vi "IKGMS.vi"(0 "delimiter (Tab)":string="\t", 1 "transpose? (no:F)":bool, 4 "format (%.3f)":string="%.2f", 5 "append to file? (new file:F)":bool, 6 "1D data":sgl[](array[numeric]) format="%.2f", 7 "2D data":sgl[][](array[numeric]) format="%.2f", 8 "file path (dialog if empty)":path) -> (3 "new file path (Not A Path if cancelled)":path)   [LabVIEW 2016]
doc: "Converts a 2D or 1D array of single-precision numbers to a text string and writes the string to a new byte stream file or appends the string to an existing file. You can optionally transpose the data. This VI opens or creates the file beforehand and closes it afterwards. You can use this VI to create a text file readable by most spreadsheet applications.\n\nfile path is the path name of the file. If file path is empty (default value) or is Not A Path, the VI displays a File dialog box from which you can select a file. Error 43 occurs if the user cancels the dialog. \n\n2D data contains the single-precision numbers the VI writes to the file if 1D data is not wired or is empty.\n\n1D data contains the single-precision numbers the VI writes to the file if this input is not empty. The VI converts the 1D array into a 2D array before transposing it and converting it to a string and writing it to the file. If transpose? is FALSE, each call to this VI creates a new line or row in the file.\n\nappend to file? Set to TRUE if you want to append the data to a existing file; you can also set it TRUE to write to a new file. Set to FALSE (default value) if you want to write the data to a new file or to replace an existing file. \n\ntranspose? Set TRUE to transpose the data before converting it to a string. The default value is FALSE.\n\nformat specifies how to convert the numbers to characters. If the format string is %.3f (default), the VI creates a string long enough to contain the number, with three digits to the right of the decimal point. If the format is %d, the VI converts the data to integer form using as many characters as necessary to contain the entire number. Refer to the discussion of format strings and the Array To Spreadsheet String function in Chapter 6, String Functions, of the LabVIEW Function Reference Manual.\n\nnew file path is the path of the file to which the VI wrote data. You can use this output to determine the path of a file that you open using dialog. new file path returns Not A Path if the user selects Cancel from the dialog box."
uses:
  ad interface/Global_SIM_switch.vi
  utilities/numrowglobal.vi
panel:
  out "NUMROWS Read":dbl format="%.2f"
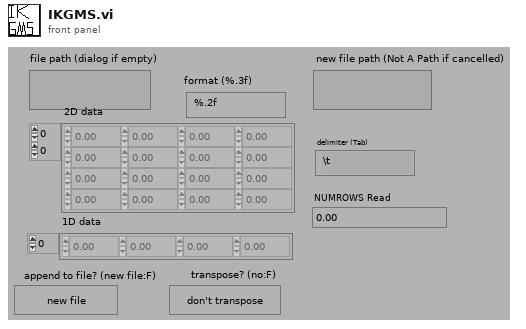
[diagram p1: front panel]
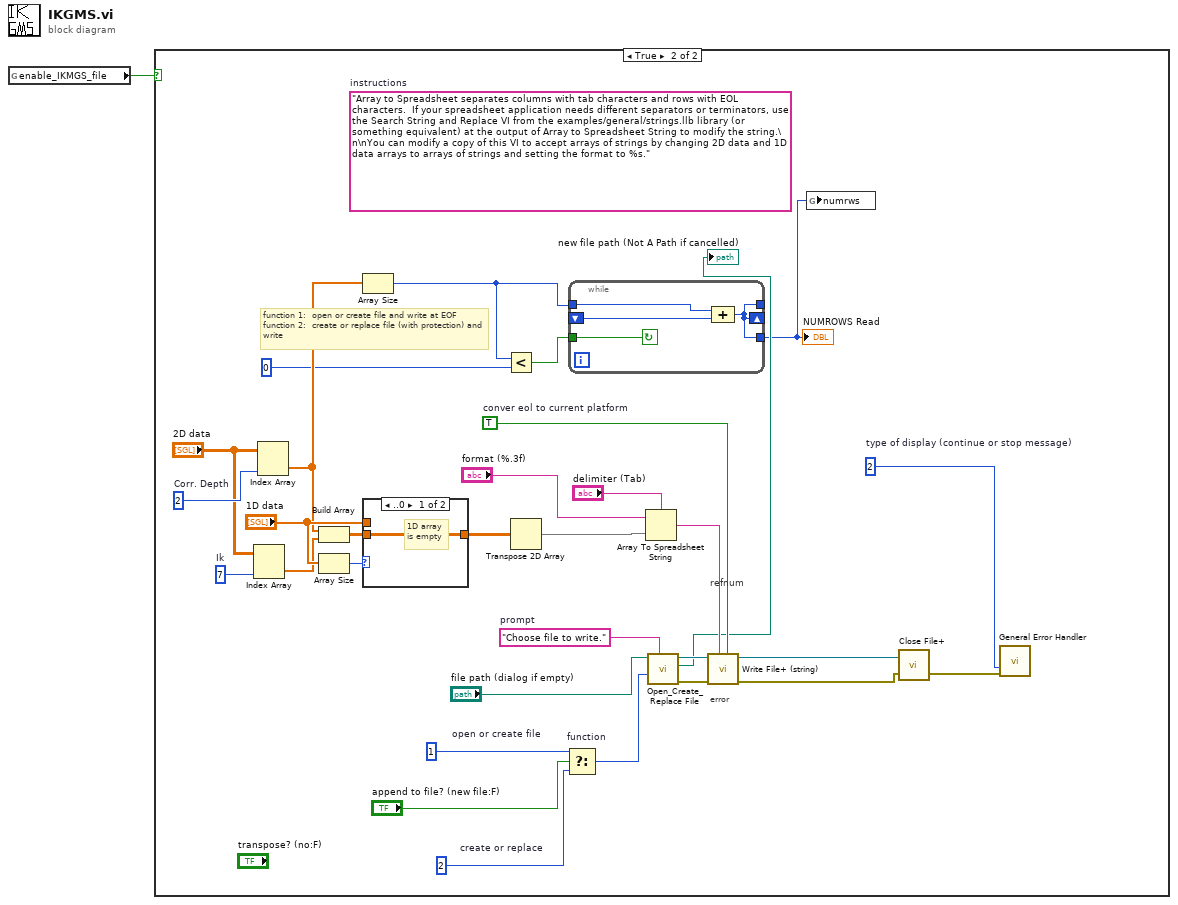
[diagram p0: block diagram]
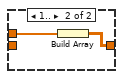
[diagram p3: hidden frame]
diagram:
  n1 = global read "Global_SIM_switch.vi" "enable_IKMGS_file"() -> (w1:bool)
  n2 = case shown="True" w1 {
    frame False {
    }
    frame True {
      w12 = 7  # Ik
      w13 = 2  # Corr. Depth
      (unwired) "Array to Spreadsheet separates columns with tab characters and rows with EOL characters.  If your spreadsheet application needs different separators or terminators, use the Search String and Replace VI from the examples/general/strings.llb library (or something equivalent) at the output of Array to Spreadsheet String to modify the string.\n\nYou can modify a copy of this VI to accept arrays of strings by changing 2D data and 1D data arrays to arrays of strings and setting the format to %s."  # instructions
      w15 = i16 2  # create or replace
      w18 = TRUE  # conver eol to current platform
      w30 = 2  # type of display (continue or stop message)
      w23 = "Choose file to write."  # prompt
      w31 = i16 1  # open or create file
      # "error"
      # "refnum"
      # "function 1:  open or create file and write at EOF\nfunction 2:  create or replace file (with protection) and write"
      n3 = Index Array(array="2D data", index (col)=w12) -> (element=w8:sgl[])  [unwired: 1 in]
      n4 = Index Array(array="2D data", index (col)=w13) -> (element=w6:sgl[])  [unwired: 1 in]
      n5 = Build Array(w6, w8) -> (w9:sgl[][])
      n6 = Array Size(array="1D data") -> (size(s)=w28:i32)
      n7 = Array Size(array=w6) -> (size(s)=w3:i32)
      n8 = case shown="..0" w28 {
        tunnel: "1D data" -> [_ w39]
        tunnel: [w37 w38] -> w11
        tunnel: w9 -> [w37 _]
        frame ..0 {
          # "1D array is empty"
        }
        frame 1.. {
          n9 = Build Array(w39) -> (w38:sgl[][])
        }
      }
      n10 = Less?(x=w3, y=0) -> (x < y?=w5:bool)
      n11 = Transpose 2D Array(2D array=w11) -> (transposed array=w10:sgl[][])
      n12 = Select "function"(t=w31, s="append to file? (new file:F)", f=w15) -> (s? t:f=w25:i16)
      n13 = while {
        tunnel: [w33] -> w2
        tunnel: w3 -> [w34]
        tunnel: [w33] -> _
        tunnel: w5 -> [w36]
        shift-left: _ -> [w35]
        shift-right: [w33] -> _
        stop <- w36 continue-if-true
        n14 = Compound Arithmetic op=ADD(w34, w35) -> (w33:i32)
      }
      "NUMROWS Read" <- w2
      n15 = Array To Spreadsheet String(delimiter (Tab)="delimiter (Tab)", array=w10, 3:"format (%.3f)") -> (spreadsheet string=w21:string)
      n16 = call <vilib>:"Open_Create_Replace File.vi"("prompt"=w23, "function (open:0)"=w25, "file path"="file path (dialog if empty)") -> ("error out"=w22:errorcluster, "new file path"=→"new file path (Not A Path if cancelled)":path, "refnum"=w17:refnum<file>)  [unwired: 5 in, 1 out]
      n17 = call <vilib>:"Write File+ (string).vi"("convert eol? (no:F)"=w18, "string"=w21, "error in (no error)"=w22, "refnum"=w17) -> ("error out"=w29:errorcluster, "dup refnum"=w20:refnum<file>)  [unwired: 3 in, 1 out]
      n18 = global write "numrowglobal.vi" "numrws"(w2) -> ()
      n19 = call <vilib>:"Close File+.vi"("error in (no error)"=w29, "refnum"=w20) -> ("error out"=w19:errorcluster)  [unwired: 3 in, 2 out]
      n20 = call <vilib>:"General Error Handler.vi"("type of dialog (OK msg:1)"=w30, "error in (no error)"=w19) -> ()  [unwired: 9 in, 5 out]
    }
  }
